vi "Channel or Section Name Valid.vi"(8 "error in (no error)":errorcluster, 10 "Name In":string, 11 "Refnum In":T1 format="%.0x") -> (0 "error out":errorcluster, 1 "Name Valid?":bool, 2 "Name Out":string, 3 "Refnum Out":T1 format="%.0x")   [LabVIEW 2018, in "Instrument Addon Scripting API.lvlib"]
uses:
  Instrument Addon Scripting API.lvlib
  <vilib>/NI Veristand/Custom Device API/Custom Device Item Ref.ctl
  <vilib>/NI Veristand/Custom Device Tools/Custom Device Utility Library/Custom Device Utility Library.lvlib
  <vilib>/NI Veristand/Custom Device API/Custom Device API.lvlib
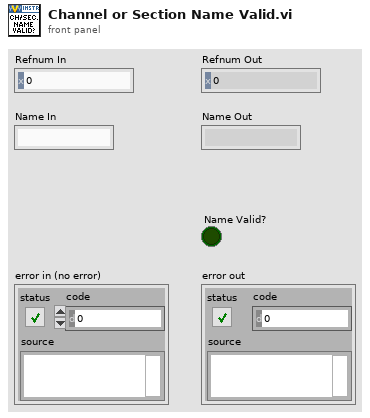
[diagram p1: front panel]
types:
  T1 = typedef "Custom Device API.lvlib/Custom Device Item Ref.ctl" = u64
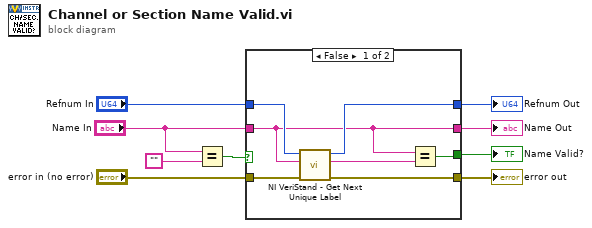
[diagram p0: block diagram]
diagram:
  n1 = Equal?(x="Name In", y="") -> (x = y?=w3:bool)
  n2 = case shown="False" w3 {
    tunnel: [w16 w18] -> w9
    tunnel: [w15 w19] -> w8
    tunnel: [w14 _] -> w7
    tunnel: "error in (no error)" -> [w13 w19]
    tunnel: "Refnum In" -> [w12 w18]
    tunnel: "Name In" -> [w10 w17]
    tunnel: [w10 w17] -> w1
    frame False {
      n3 = call <vilib>:"NI VeriStand - Get Next Unique Label.vi"("error in (no error)"=w13, "Label"=w10, "Parent Ref in"=w12) -> ("error out"=w15:errorcluster, "Label out"=w11:string, "Parent Ref dup"=w16:T1)  [unwired: 5 in, 1 out]
      n4 = Equal?(x=w10, y=w11) -> (x = y?=w14:bool)
    }
    frame True {
    }
  }
  "Refnum Out" <- w9
  "error out" <- w8
  "Name Valid?" <- w7
  "Name Out" <- w1
